vi "Configure.vi"(8 "error in (no error)":errorcluster, 11 "navX - Base in":refnum<class "navX - Base.lvclass">) -> (0 "error out":errorcluster, 3 "navX - Base out":refnum<class "navX - Base.lvclass">)   [LabVIEW 2015, in "navX Library v3.lvlib" / "navX - Base.lvclass"]
uses:
  navX - Base.lvclass
  navX - Base.lvclass/navX - Base.ctl
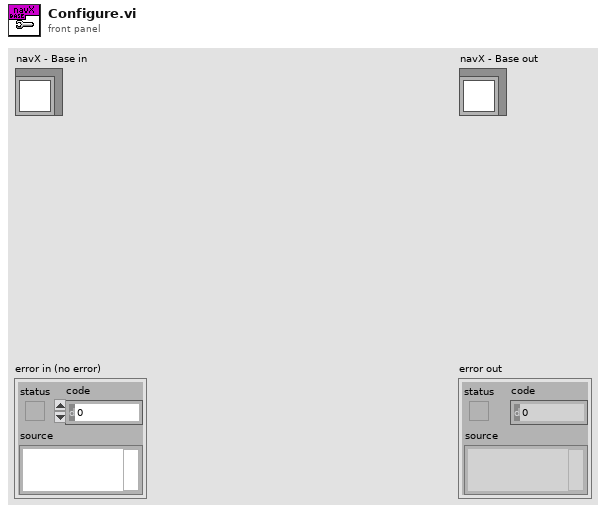
[diagram p1: front panel]
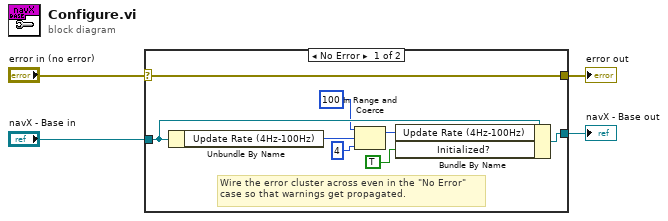
[diagram p0: block diagram]
diagram:
  n1 = case shown="No Error" "error in (no error)" {
    selector: "error in (no error)" -> [w12 w14]
    tunnel: [w12 w14] -> w3
    tunnel: [w11 w13] -> w1
    tunnel: "navX - Base in" -> [w10 w13]
    frame No Error {
      # "Wire the error cluster across even in the \"No Error\"\ncase so that warnings get propagated."
      n2 = Unbundle By Name(w10) -> ("Update Rate (4Hz-100Hz)"=w8:u8)
      n3 = In Range and Coerce(upper limit=u8 100, x=w8, lower limit=u8 4) -> (coerced(x)=w7:u8)  [unwired: 1 out]
      n4 = Bundle By Name(cluster=w10, "Update Rate (4Hz-100Hz)"=w7, "Initialized?"=TRUE) -> (w11:refnum<class "navX - Base.lvclass">)
    }
    frame Error {
    }
  }
  "error out" <- w3
  "navX - Base out" <- w1
